vi "Read Data Rate.vi"(8 "error in (no error)":errorcluster, 11 "Daqmx Module configuration in":refnum<class "DAQmx Module Configuration.lvclass">) -> (0 "error out":errorcluster, 2 "Rate":dbl, 3 "Daqmx Module configuration out":refnum<class "DAQmx Module Configuration.lvclass">)   [LabVIEW 2014, in "DAQmx Module Configuration.lvclass"]
uses:
  DAQmx Module Configuration.lvclass
  DAQmx Module Configuration.lvclass/DAQmx Module Configuration.ctl
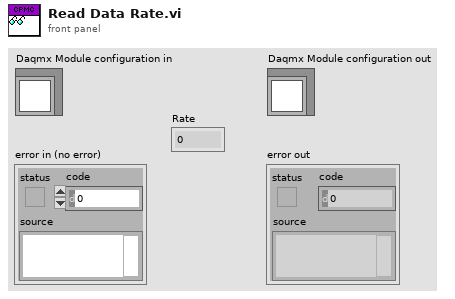
[diagram p1: front panel]
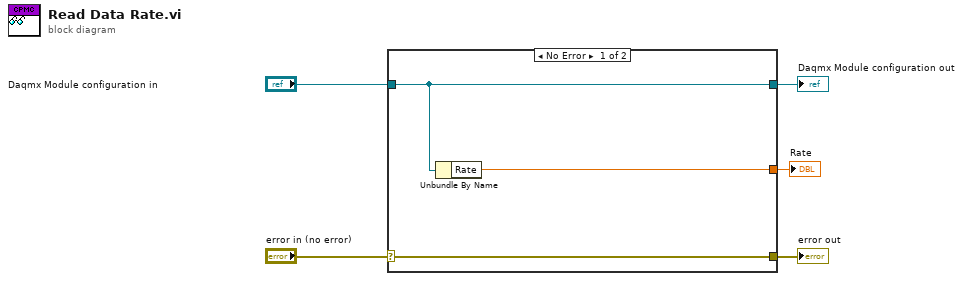
[diagram p0: block diagram]
diagram:
  n1 = case shown="No Error" "error in (no error)" {
    selector: "error in (no error)" -> [w8 w9]
    tunnel: [w8 w9] -> w4
    tunnel: [w7 w10] -> w2
    tunnel: "Daqmx Module configuration in" -> [w7 w10]
    tunnel: [w6 _] -> w1
    frame No Error {
      n2 = Unbundle By Name(w7) -> ("Rate"=w6:dbl)
    }
    frame Error {
    }
  }
  "error out" <- w4
  "Daqmx Module configuration out" <- w2
  "Rate" <- w1
